vi "Error - Fire Error.vi"(8 "error in (no error)":errorcluster, 10 "Error Type":T1, 11 "View Model":T2) -> (0 "error out":errorcluster, 3 "View Model":T2)   [LabVIEW 2017]
doc: "Generates Error User Event with parameters (Variant)."
uses:
  View Model/Controls/View Model.ctl
  Configuration/Controls/Config Model.ctl
  Configuration/Controls/Config Data.ctl
  Controls/Error Model.ctl
  Controls/Error Data.ctl
  Controls/Error Type.ctl
  View Model/Controls/Shared Model.ctl
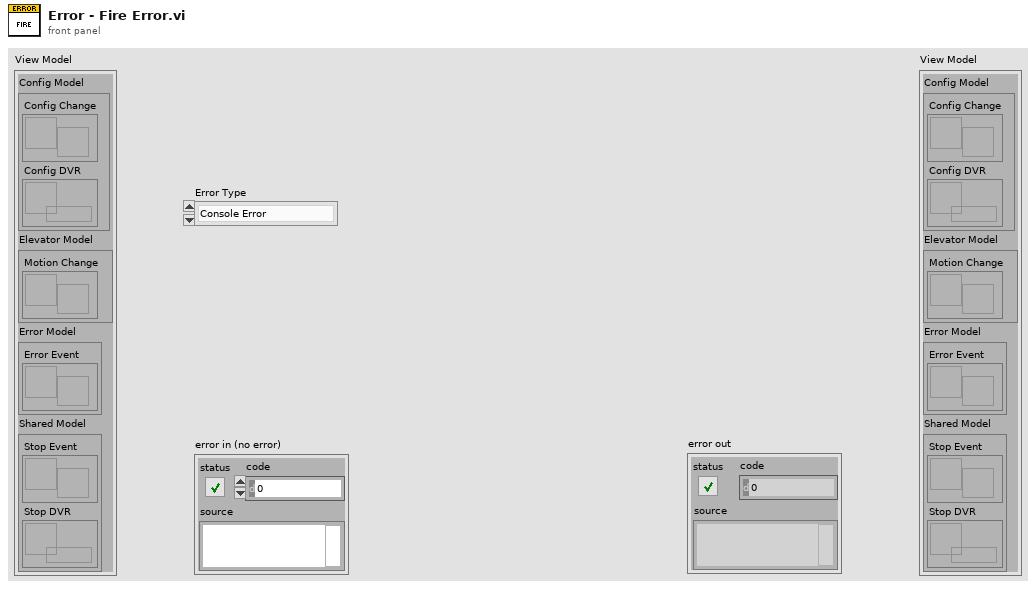
[diagram p1: front panel]
types:
  T1 = typedef "Error Type.ctl" = enum16{"Console Error", "Sensor Interface IO Error", "Process Step Error"}
  T2 = typedef "View Model.ctl" = cluster{"Config Model":T3, "Elevator Model":cluster{"Motion Change":refnum<user-event>}, "Error Model":T4, "Shared Model":T5}
  T3 = typedef "Config Model.ctl" = cluster{"Config Change":refnum<user-event>, "Config DVR":refnum<data-value>}
  T4 = typedef "Error Model.ctl" = cluster{"Error Event":refnum<user-event>}
  T5 = typedef "Shared Model.ctl" = cluster{"Stop Event":refnum<user-event>, "Stop DVR":refnum<data-value>}
  T6 = typedef "Error Data.ctl" = cluster{"Error Type":T1, "Variant":variant}
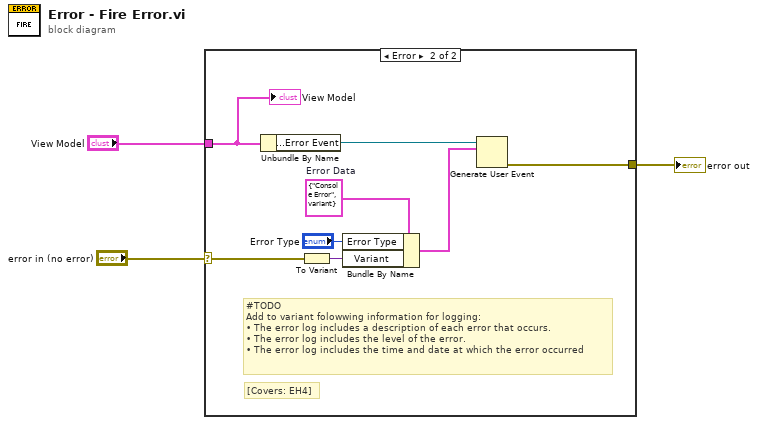
[diagram p0: block diagram]
diagram:
  n1 = case shown="Error" "error in (no error)" {
    selector: "error in (no error)" -> [w4 w7]
    tunnel: "View Model" -> [_ w11]
    tunnel: [w4 w5] -> w1
    frame No Error {
    }
    frame Error {
      w10 = T6 {"Error Type"=enum."Console Error", "Variant"=variant}  # Error Data
      # "[Covers: EH4]"
      # "#TODO\nAdd to variant folowwing information for logging:\n• The error log includes a description of each error that occurs.\n• The error log includes the level of the error.\n• The error log includes the time and date at which the error occurred"
      n2 = Unbundle By Name(w11) -> ("Error Model.Error Event"=w12:refnum<user-event>)
      n3 = To Variant(anything=w7) -> (Variant=w6:variant)
      n4 = Bundle By Name(cluster=w10, "Error Type"="Error Type", "Variant"=w6) -> (w8:T6)
      n5 = Generate User Event(user event=w12, event data cluster=w8) -> (error out=w5:errorcluster)  [unwired: 2 in, 1 out]
      "View Model" <- w11
    }
  }
  "error out" <- w1
